vi "Launcher Data Analysis.vi"() -> ()   [LabVIEW 2023, in "Data Analysis.lvlib"]
uses:
  Data Analysis.lvlib
  Post Analysis/Post Analysis.lvclass
  <vilib>/ActorFramework/Actor/Actor.lvclass
panel:
  out "version":string
  # "LTT Data Analyser"
  # "Initializing...."
  # "Designed and Developed by"
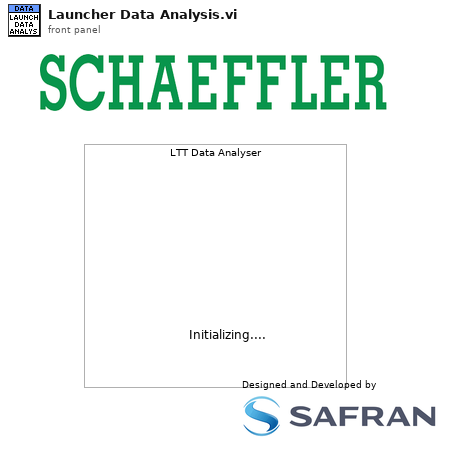
[diagram p1: front panel]
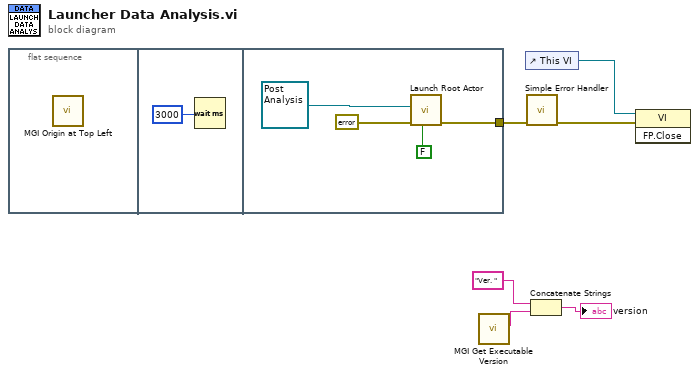
[diagram p0: block diagram]
diagram:
  n1 = flat-sequence {
    tunnel: [w8] -> w4
    frame #0 {
      n2 = call <userlib>:"MGI Origin at Top Left.vi"() -> ()  [unwired: 9 in, 2 out]
    }
    frame #1 {
      n3 = Wait (ms)(milliseconds to wait=u32 3000) -> ()  [unwired: 1 out]
    }
    frame #2 {
      n4 = call <vilib>:"Launch Root Actor.vi"("Open Actor Core front panel? (F)"=FALSE, "error in (no error)"=errorcluster {"status"=FALSE, "code"=0, "source"=""}, "Actor"=refnum<class "Post Analysis.lvclass"> refnum ("Data Analysis.lvlib:Post Analysis.lvlib:Post Analysis.lvclass")) -> ("error out"=w8:errorcluster)  [unwired: 7 in, 1 out]
    }
  }
  n5 = call <userlib>:"MGI Get Executable Version.vi"() -> ("Version"=w1:string)  [unwired: 7 in]
  n6 = control-ref of="This VI"() -> (w6:refnum<vi>)
  n7 = call <vilib>:"Simple Error Handler.vi"("error in (no error)"=w4) -> ("error out"=w5:errorcluster)  [unwired: 4 in, 4 out]
  n8 = Concatenate Strings("Ver. " ("string"), w1) -> (→"version":string)
  n9 = invoke class="VI" method="FP.Close"(reference=w6, error in=w5) -> ()  [unwired: 1 in, 3 out]
